vi "InFamily.vi"(10 "String 2":string, 11 "String 1":string) -> (3 "Family?":bool)   [LabVIEW 2022 SP3]
uses:
  <userlib>/_OpenG.lib/file/file.llb/Strip Path Extension - String__ogtk.vi
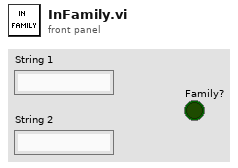
[diagram p1: front panel]
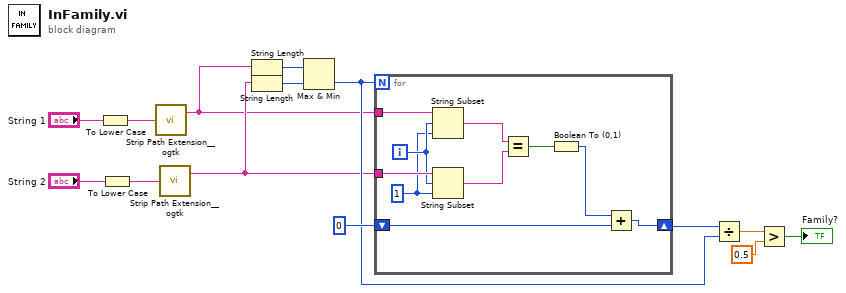
[diagram p0: block diagram]
diagram:
  n1 = To Lower Case(string="String 1") -> (all lower case string=w2:string)
  n2 = To Lower Case(string="String 2") -> (all lower case string=w4:string)
  n3 = call-poly <userlib>:"Strip Path Extension__ogtk.vi"("path"=w2) -> ("root"=w1:string)  [unwired: 1 out]
  n4 = call-poly <userlib>:"Strip Path Extension__ogtk.vi"("path"=w4) -> ("root"=w3:string)  [unwired: 1 out]
  n5 = String Length(string=w1) -> (length=w14:i32)
  n6 = String Length(string=w3) -> (length=w13:i32)
  n7 = Max & Min(x=w14, y=w13) -> (min(x,y)=w10:i32)  [unwired: 1 out]
  n8 = for {
    N: w10 -> [_]
    tunnel: w1 -> [w24]
    tunnel: w3 -> [w23]
    shift-right: [w17] -> w11
    shift-left: 0 -> [w16]
    i -> [w22]
    w21 = 1 ("length (rest)")
    n9 = String Subset(string=w24, offset (0)=w22, length (rest)=w21) -> (substring=w20:string)
    n10 = String Subset(string=w23, offset (0)=w22, length (rest)=w21) -> (substring=w19:string)
    n11 = Equal?(x=w20, y=w19) -> (x = y?=w18:bool)
    n12 = Boolean To (0,1)(Boolean=w18) -> (0, 1=w15:i16)
    n13 = Add(x=w15, y=w16) -> (x+y=w17:i32)
  }
  n14 = Divide(x=w11, y=w10) -> (x/y=w7:dbl)
  n15 = Greater?(x=w7, y=0.5) -> (0:→"Family?":bool)
